vi "Write Headers.vi"(8 "AKLH Today Dirs":path[](array[path]), 9 "Data Log Dirs":path[](array[path]), 10 "Controller Type":string, 11 "App Config":T1={"Location"="", "Profiles Path"=path "", "Current Profile"="", "CA Number"="", "Cycles Completed"=0, "Controller Type:"=enum."Kuhnke", "Stagger Time (ms)"=0, "Tank 1 Fuel"="", "Tank 2 Fuel"="", "Serial Numbers"={"Position 1 SN"="", "Position 2 SN"="", "Poaition 3 SN"="", "Position 4 SN"="", "Position 5 SN"="", "Position 6 SN"=""}, "Pumps Present"={"Pump 1"=FALSE, "Pump 2"=FALSE, "Pump 3"=FALSE, "Pump 4"=FALSE, "Pump 5"=FALSE, "Pump 6"=FALSE}, "VoltCtrlRef"="", "VoltageSelect"=FALSE, "Watlow Present"=FALSE, "Temp 1"=0.0, "Temp 2"=0.0, "V_Run PI?"=FALSE, "Voltage Limits"={"V_Step"=1e-05, "V_CmdMax"=0.0, "V_CmdMin"=0.0}, "Voltage Far PI"={"V_FarSlew"=10.0, "V_FarKp"=0.0, "V_FarKi"=0.0}, "Voltage Mid PI"={"V_MidSlew"=10.0, "V_MidKp"=0.0, "V_MidKi"=0.0}, "Voltage Close PI"={"V_CloseSlew"=10.0, "V_CloseKp"=0.0, "V_CloseKi"=0.0}, "Voltage Scale"={"V_FFm"=0.0, "V_FFb"=0.0}, "Voltage Cutoffs"={"V_MidCutoff"=0.0, "V_CloseCutoff"=0.0}, "Pressure Scale"={"Pres_FFm"=1e-05, "Pres_FFb"=0.0}, "Temp Format"=0, "Temp Tolerance"=0.0, "Target Voltage"=0.0, "Target Pressure"=0.0, "Data Log Init"={"Data Path"=path "", "Data Log Rate (S/s)"=0, "AKLH Rate (Hours/S)"=0.0, "Sync Time Offset (min)"=0, "IP Last 3"=0, "WebDAV IP"=""}, "Email Handler IP"="", "ADC Check"=FALSE, "3 Pump Tank"=FALSE, "Cycle Threshold:"=3.0, "Cycle Pts to Avg:"=3, "Anomaly Threshold:"=3.0, "Normal Steps:"=3, "Step Threshold:"=3.0, "Network Drive IP"="", "Network Drive Password"="", "Bank 1 Offset"=0.0, "Bank 2 Offset"=0.0} {"Bank 2 Offset" min=0.0 max=999999.0 step=1.0; "Bank 1 Offset" min=0.0 max=999999.0 step=1.0; "Step Threshold:" min=0.0 max=999999.0 step=1.0; "Normal Steps:" max=999999 step=1; "Anomaly Threshold:" min=0.0 max=999999.0 step=1.0; "Cycle Pts to Avg:" max=999999 step=1; "Cycle Threshold:" min=0.0 max=999999.0 step=1.0}) -> (2 "AKLH Today Header Paths":path[](array[path]), 3 "Data Log Header Paths":path[](array[path]))   [LabVIEW 2018]
uses:
  Type Defs/App Config.ctl
  Type Defs/Controller Names.ctl
  Data Log Init.ctl
  <vilib>/Utility/file.llb/Write To Spreadsheet File (string).vi
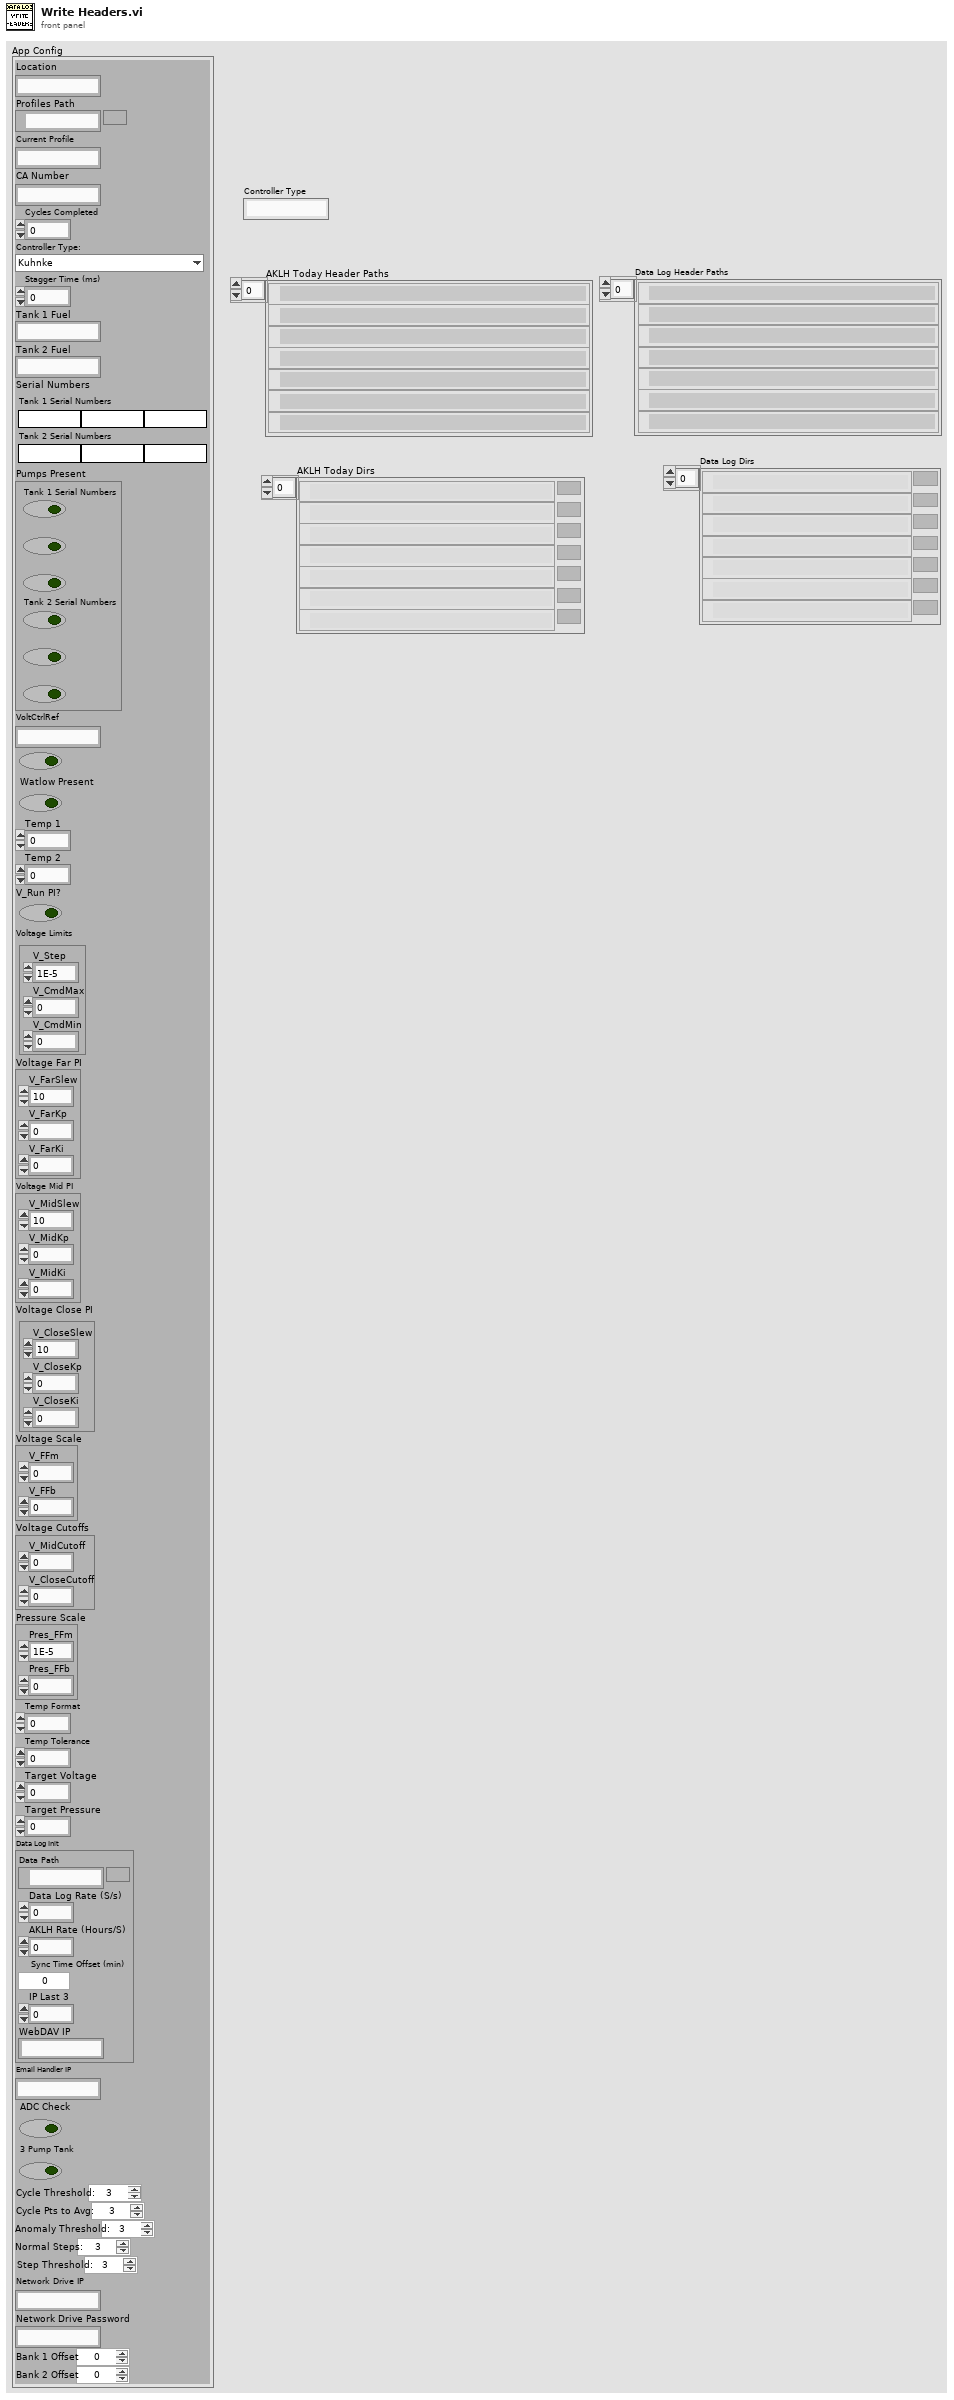
[diagram p1: front panel]
types:
  T1 = typedef "App Config.ctl" = cluster{"Location":string, "Profiles Path":path, "Current Profile":string, "CA Number":string, "Cycles Completed":u32, "Controller Type:":T2, "Stagger Time (ms)":i32, "Tank 1 Fuel":string, "Tank 2 Fuel":string, "Serial Numbers":cluster{"Position 1 SN":string, "Position 2 SN":string, "Poaition 3 SN":string, "Position 4 SN":string, "Position 5 SN":string, "Position 6 SN":string}, "Pumps Present":cluster{"Pump 1":bool, "Pump 2":bool, "Pump 3":bool, "Pump 4":bool, "Pump 5":bool, "Pump 6":bool}, "VoltCtrlRef":string, "VoltageSelect":bool, "Watlow Present":bool, "Temp 1":dbl, "Temp 2":dbl, "V_Run PI?":bool, "Voltage Limits":cluster{"V_Step":dbl, "V_CmdMax":dbl, "V_CmdMin":dbl}, "Voltage Far PI":cluster{"V_FarSlew":dbl, "V_FarKp":dbl, "V_FarKi":dbl}, "Voltage Mid PI":cluster{"V_MidSlew":dbl, "V_MidKp":dbl, "V_MidKi":dbl}, "Voltage Close PI":cluster{"V_CloseSlew":dbl, "V_CloseKp":dbl, "V_CloseKi":dbl}, "Voltage Scale":cluster{"V_FFm":dbl, "V_FFb":dbl}, "Voltage Cutoffs":cluster{"V_MidCutoff":dbl, "V_CloseCutoff":dbl}, "Pressure Scale":cluster{"Pres_FFm":dbl, "Pres_FFb":dbl}, "Temp Format":i32, "Temp Tolerance":dbl, "Target Voltage":dbl, "Target Pressure":dbl, "Data Log Init":T3, "Email Handler IP":string, "ADC Check":bool, "3 Pump Tank":bool, "Cycle Threshold:":dbl, "Cycle Pts to Avg:":i32, "Anomaly Threshold:":dbl, "Normal Steps:":u32, "Step Threshold:":dbl, "Network Drive IP":string, "Network Drive Password":string, "Bank 1 Offset":dbl, "Bank 2 Offset":dbl}
  T2 = typedef "Controller Names.ctl" = enum16{"Kuhnke", "Helbako BLDC", "Conti", "Hella BLDC OL PWM", "Hella BLDC Turbine OL PWM", "Hella BLDC Pressure", "Helbako (old)", "TI PWM", "PSA", "Hella Gas", "Hella Diesel", "8 Comm", "10 Comm", "8 Comm Hella", "10 Comm Hella", "8 Comm Omron", "10 Comm Omron", "8 Comm Nissan", "10 Comm Nissan"}
  T3 = typedef "Data Log Init.ctl" = cluster{"Data Path":path, "Data Log Rate (S/s)":u32, "AKLH Rate (Hours/S)":dbl, "Sync Time Offset (min)":i32, "IP Last 3":i32, "WebDAV IP":string}
  T4 = cluster{"Position 1 SN":string, "Position 2 SN":string, "Poaition 3 SN":string, "Position 4 SN":string, "Position 5 SN":string, "Position 6 SN":string}
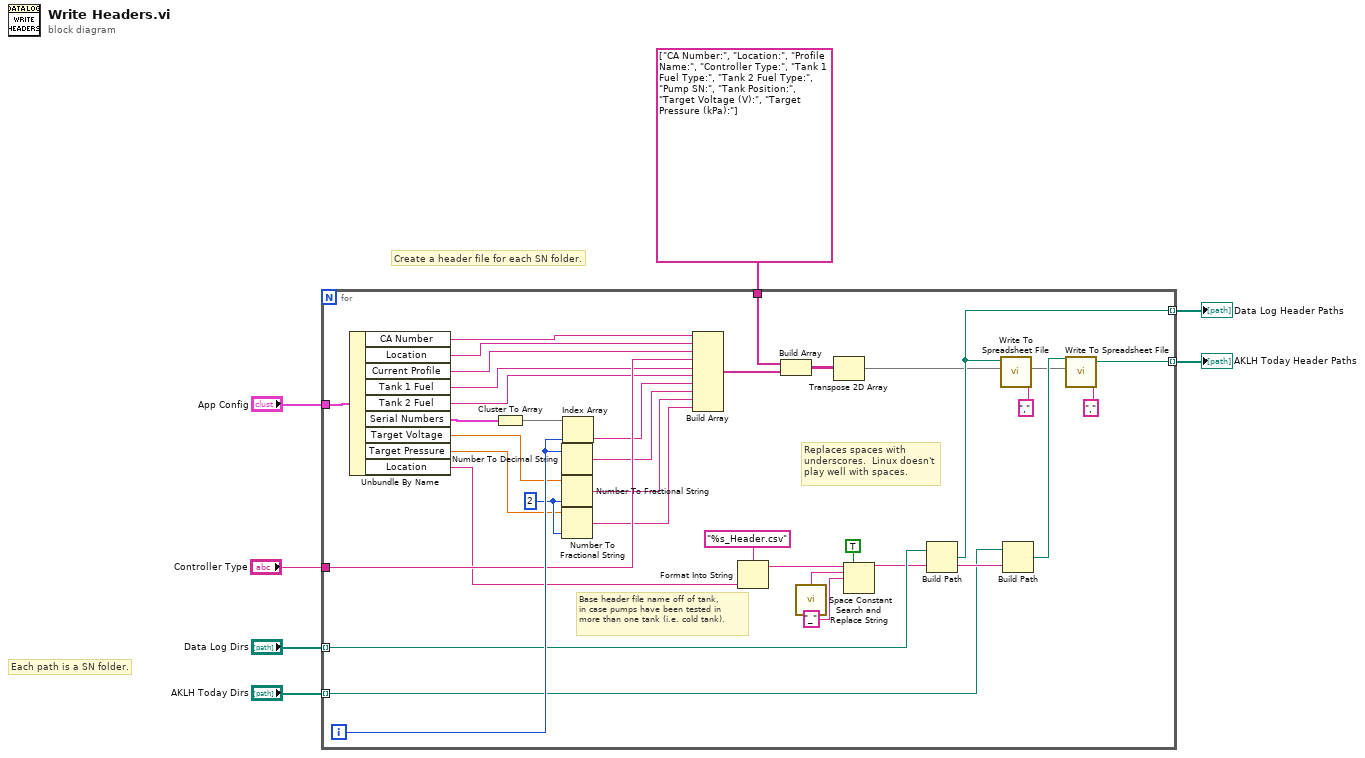
[diagram p0: block diagram]
diagram:
  # "Create a header file for each SN folder."
  # "Each path is a SN folder."
  n1 = for {
    tunnel: "Data Log Dirs" -> [w21] mode=indexing
    tunnel: "AKLH Today Dirs" -> [w19] mode=indexing
    tunnel: "App Config" -> [w42]
    tunnel: "Controller Type" -> [w35]
    tunnel: string[] ["CA Number:", "Location:", "Profile Name:", "Controller Type:", "Tank 1 Fuel Type:", "Tank 2 Fuel Type:", "Pump SN:", "Tank Position:", "Target Voltage (V):", "Target Pressure (kPa):"] -> [w30]
    tunnel: [w15] -> w2 mode=indexing
    tunnel: [w14] -> w1 mode=indexing
    i -> [w39]
    w12 = i16 2 ("precision (6)")
    # "Base header file name off of tank,\nin case pumps have been tested in\nmore than one tank (i.e. cold tank)."
    # "Replaces spaces with\nunderscores.  Linux doesn't\nplay well with spaces."
    n2 = Unbundle By Name(w42) -> ("CA Number"=w38:string, "Location"=w37:string, "Current Profile"=w36:string, "Tank 1 Fuel"=w34:string, "Tank 2 Fuel"=w33:string, "Serial Numbers"=w41:T4, "Target Voltage"=w13:dbl, "Target Pressure"=w11:dbl, "Location"=w27:string)
    n3 = Cluster To Array(cluster=w41) -> (array=w40:string[])
    n4 = Number To Decimal String(number=w39) -> (decimal integer string=w31:string)  [unwired: 1 in]
    n5 = Number To Fractional String(number=w13, precision (6)=w12) -> (F-format string=w10:string)  [unwired: 2 in]
    n6 = Number To Fractional String(number=w11, precision (6)=w12) -> (F-format string=w9:string)  [unwired: 2 in]
    n7 = Index Array(array=w40, index=w39) -> (element=w32:string)
    n8 = Build Array(w38, w37, w36, w35, w34, w33, w32, w31, w10, w9) -> (w29:string[])
    n9 = Format Into String(format string="%s_Header.csv", w27) -> (resulting string=w24:string)  [unwired: 2 in, 1 out]
    n10 = Build Array(w30, w29) -> (w16:string[][])
    n11 = call <vilib>:"Space Constant.vi"() -> ("String"=w23:string)
    n12 = Transpose 2D Array(2D array=w16) -> (transposed array=w8:string[][])
    n13 = Search and Replace String(replace all?=TRUE ("replace all? (F)"), input string=w24, search string=w23, replace string="_" ("replace string (\"\")")) -> (result string=w20:string)  [unwired: 4 in, 3 out]
    n14 = Build Path(base path=w21, name or relative path=w20) -> (appended path=w15:path)
    n15 = call-poly <vilib>:"Write To Spreadsheet File.vi"("delimiter (\\t)"="," ("delimiter (\\t)"), "2D data"=w8, "file path (dialog if empty)"=w15) -> ()  [unwired: 5 in, 1 out]
    n16 = Build Path(base path=w19, name or relative path=w20) -> (appended path=w17:path)
    n17 = call-poly <vilib>:"Write To Spreadsheet File.vi"("delimiter (\\t)"="," ("delimiter (\\t)"), "2D data"=w8, "file path (dialog if empty)"=w17) -> ("new file path (Not A Path if cancelled)"=w14:path)  [unwired: 5 in]
  }
  "Data Log Header Paths" <- w2
  "AKLH Today Header Paths" <- w1
